vi "AVS_GetList.vi"(0 "ListSizeInput":u32, 7 "RequiredSizeInput":u32, 11 "ListInpit":u8[](array[numeric])) -> (4 "ListSizeOutput":u32, 8 "RequiredSizeOutput":u32, 15 "List Output":u8[](array[numeric]))   [LabVIEW 2020]
uses:
  AvaSpecX64-DLL_9.4/avaspecx64.dll
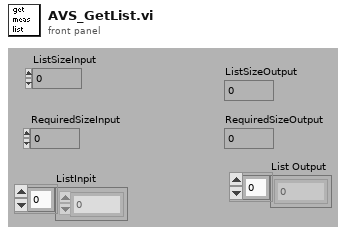
[diagram p1: front panel]
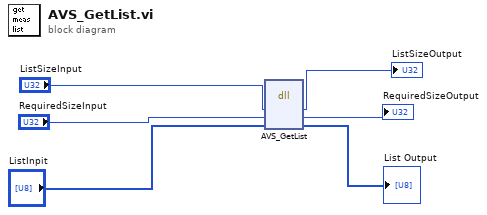
[diagram p0: block diagram]
diagram:
  n1 = dll-call lib="C:/AvaSpecX64-DLL_9.4/avaspecx64.dll" fn="AVS_GetList"("a_ListSize"="ListSizeInput", "a_pRequiredSize"="RequiredSizeInput", "a_pList"="ListInpit") -> ("a_ListSize"=→"ListSizeOutput":u32, "a_pRequiredSize"=→"RequiredSizeOutput":u32, "a_pList"=→"List Output":u8[])  [unwired: 4 in, 2 out]
